vi "2D Array of Python Strings to Python List.vi"(8 "error in (no error)":errorcluster, 10 "Array of Python Strings":string[][](array[string])) -> (0 "error out":errorcluster, 2 "Python List":string)   [LabVIEW 2020, in "jki_python_data_tools.lvlib"]
uses:
  jki_python_data_tools.lvlib
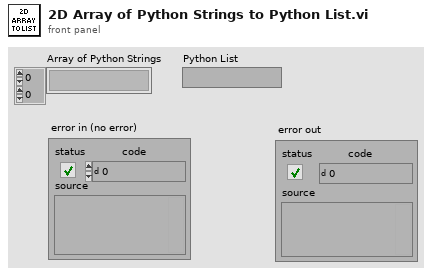
[diagram p1: front panel]
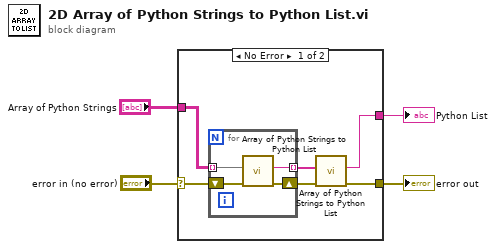
[diagram p0: block diagram]
diagram:
  n1 = case shown="No Error" "error in (no error)" {
    selector: "error in (no error)" -> [w10 w15]
    tunnel: [w6 _] -> w4
    tunnel: "Array of Python Strings" -> [w9 _]
    tunnel: [w7 w15] -> w1
    frame No Error {
      n2 = for {
        tunnel: w9 -> [w12] mode=indexing
        tunnel: [w11] -> w5 mode=indexing
        shift-right: [w13] -> w8
        shift-left: w10 -> [w14]
        n3 = call "Array of Python Strings to Python List.vi"("error in (no error)"=w14, "Array of Python Strings"=w12) -> ("error out"=w13:errorcluster, "Python List"=w11:string)  [unwired: 8 in]
      }
      n4 = call "Array of Python Strings to Python List.vi"("error in (no error)"=w8, "Array of Python Strings"=w5) -> ("error out"=w7:errorcluster, "Python List"=w6:string)  [unwired: 8 in]
    }
    frame Error {
    }
  }
  "Python List" <- w4
  "error out" <- w1
